vi "niRFUtil FTW FIR Filter (complex wfm).vi"(1 "Filter":T1 {"y" min=0 max=127 format="%.2f"; "dx" format="%^.2e"; "x0" format="%^.2e"}, 2 "Waveform In":T3 {"y" format="%.2f"; "dx" format="%^.2e"; "x0" format="%^.2e"}) -> (0 "Waveform Out":T3 {"y" format="%.2f"; "dx" format="%^.2e"; "x0" format="%^.2e"})   [LabVIEW 2016, in "niRFUtil.lvlib"]
doc: "(c) Copyright 2006, National Instruments, Inc. This VI may not be duplicated, sold, or distributed without written consent from National Instruments."
uses:
  niRFUtil.lvlib
  Includes/niRFUtil INC Complex Waveform.ctl
  Includes/niRFUtil INC Complex Array.ctl
  Includes/niRFUtil INC Real Waveform.ctl
  Includes/niRFUtil INC Real Array.ctl
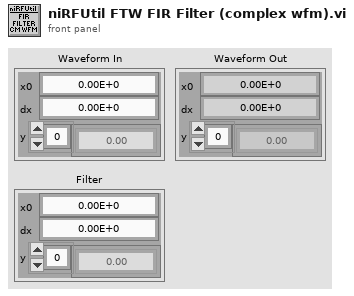
[diagram p1: front panel]
types:
  T1 = typedef "niRFUtil.lvlib/niRFUtil INC Real Waveform.ctl" = cluster{"x0":dbl, "dx":dbl, "y":T2}
  T2 = typedef "niRFUtil.lvlib/niRFUtil INC Real Array.ctl" = sgl[]
  T3 = typedef "niRFUtil.lvlib/niRFUtil INC Complex Waveform.ctl" = cluster{"x0":dbl, "dx":dbl, "y":T4}
  T4 = typedef "niRFUtil.lvlib/niRFUtil INC Complex Array.ctl" = csg[]
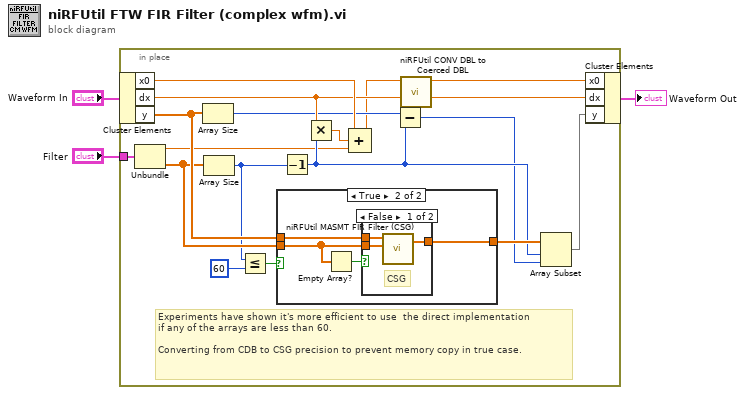
[diagram p0: block diagram]
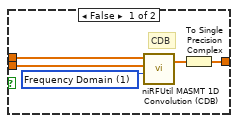
[diagram p2: hidden frame]
diagram:
  n1 = in-place {
    in-place-border: "Filter" -> [w12]
    # "Experiments have shown it's more efficient to use  the direct implementation\nif any of the arrays are less than 60. \n\nConverting from CDB to CSG precision to prevent memory copy in true case."
    n2 = in-place-cluster #1("Waveform In") -> ("x0"=w19:dbl, "dx"=w17:dbl, "y"=w18:T4)
    n3 = Unbundle(w12) -> ("x0"=w11:dbl, "y"=w9:T2)  [unwired: 1 out]
    n4 = Array Size(array=w18) -> (size(s)=w13:i32)
    n5 = Array Size(array=w9) -> (size(s)=w7:i32)
    n6 = Less Or Equal?(x=w7, y=60) -> (x <= y?=w8:bool)
    n7 = case shown="True" w8 {
      tunnel: [w21 w29] -> w20
      tunnel: w18 -> [w23 w28]
      tunnel: w9 -> [w24 w26]
      frame False {
        w25 = 1 items=["Direct", "Frequency Domain"] ("algorithm")
        # "CDB"
        n8 = call "niRFUtil MASMT 1D Convolution (CDB).vi"("algorithm"=w25, "Y"=w24, "X"=w23) -> ("X * Y"=w22:cdb[])  [unwired: 7 in, 1 out]
        n9 = To Single Precision Complex(1:w22) -> (0:w21:csg[])
      }
      frame True {
        n10 = Empty Array?(array=w26) -> (empty?=w27:bool)
        n11 = case shown="False" w27 {
          tunnel: [w32 _] -> w29
          tunnel: w28 -> [w31 _]
          tunnel: w26 -> [w30 _]
          frame False {
            # "CSG"
            n12 = call "niRFUtil MASMT FIR Filter (CSG).vi"("FIR Coefficients"=w30, "X"=w31) -> ("Filtered X"=w32:csg[])  [unwired: 8 in, 1 out]
          }
          frame True {
          }
        }
      }
    }
    n13 = Decrement(x=w7) -> (x-1=w15:i32)
    n14 = Multiply(x=w17, y=w15) -> (x*y=w16:dbl)
    n15 = Compound Arithmetic op=ADD(w19, w16, w11) -> (w5:dbl)
    n16 = Subtract(x=w13, y=w15) -> (x-y=w14:i32)
    n17 = call "niRFUtil CONV DBL to Coerced DBL.vi"("Numeric In (DBL)"=w5) -> ("Coerced Numeric Out (DBL)"=w4:dbl)  [unwired: 10 in]
    n18 = Array Subset(array=w20, index=w15, length=w14) -> (w10:csg[])
    n19 = in-place-cluster #1("x0"=w4, "dx"=w17, "y"=w10) -> (→"Waveform Out":T3)
  }
